vi "Create class folders.vi"() -> ()   [LabVIEW 2015]
panel:
  in  "Class Path":path
  in  "Host":bool=TRUE
  in  "Project Path":path
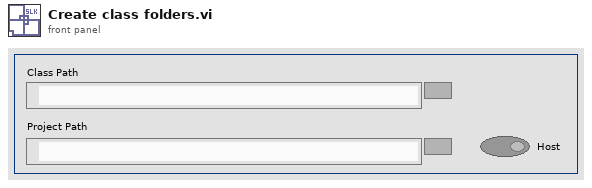
[diagram p1: front panel]
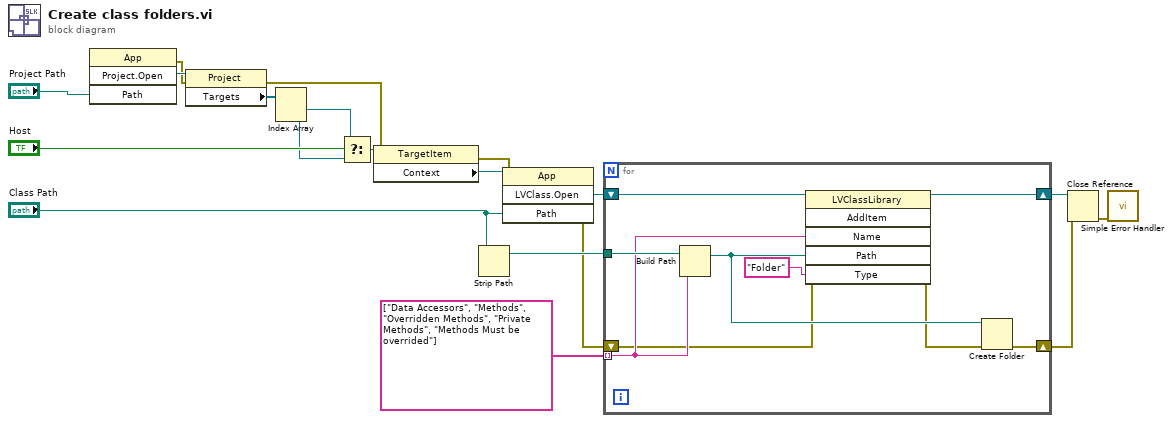
[diagram p0: block diagram]
diagram:
  n1 = invoke class="App" method="Project.Open"("Path"="Project Path") -> (error out=w6:errorcluster, "Project:Open"=w18:refnum<vi>)  [unwired: 3 in, 2 out]
  n2 = property class="Project"(reference=w18, error in=w6) -> (error out=w5:errorcluster, "Targets"=w17:refnum<vi>[])  [unwired: 1 out]
  n3 = Index Array(array=w17) -> (element #1=w15:refnum<vi>, element #2=w14:refnum<vi>)  [unwired: 2 in]
  n4 = Select(t=w15, s="Host", f=w14) -> (s? t:f=w13:refnum<vi>)
  n5 = property class="TargetItem"(reference=w13, error in=w5) -> (error out=w4:errorcluster, "Context"=w12:refnum<vi>)  [unwired: 1 out]
  n6 = Strip Path(path="Class Path") -> (stripped path=w8:path)  [unwired: 1 out]
  n7 = invoke class="App" method="LVClass.Open"(reference=w12, error in=w4, "Path"="Class Path") -> (error out=w3:errorcluster, "LVClass.Open"=w11:refnum<vi>)  [unwired: 1 in, 2 out]
  n8 = for {
    tunnel: string[] ["Data Accessors", "Methods", "Overridden Methods", "Private Methods", "Methods Must be overrided"] ("folder Names") -> [w25] mode=indexing
    tunnel: w8 -> [w26]
    shift-right: [w24] -> w7
    shift-left: w11 -> [w28]
    shift-right: [w21] -> w2
    shift-left: w3 -> [w20]
    n9 = Build Path(base path=w26, name or relative path=w25) -> (appended path=w23:path)
    n10 = invoke class="LVClassLibrary" method="AddItem"(reference=w28, error in=w20, "Name"=w25, "Path"=w23, "Type"="Folder" ("类型")) -> (reference out=w24:refnum<vi>, error out=w22:errorcluster)  [unwired: 1 in, 4 out]
    n11 = Create Folder(path (use dialog)=w23, error in=w22) -> (error out=w21:errorcluster)  [unwired: 1 in, 2 out]
  }
  n12 = Close Reference(reference=w7, error in (no error)=w2) -> (error out=w1:errorcluster)
  n13 = call <vilib>:"Simple Error Handler.vi"("error in (no error)"=w1) -> ()  [unwired: 4 in, 5 out]
